vi "Vector Unique Values.vi"(1 "array in":dbl[](array[numeric])) -> (0 "uniques out":dbl[](array[numeric]))   [LabVIEW 2020]
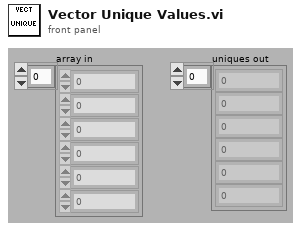
[diagram p1: front panel]
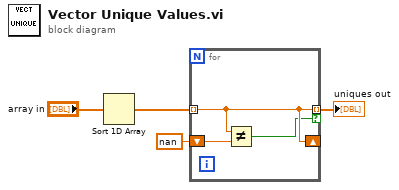
[diagram p0: block diagram]
diagram:
  n1 = Sort 1D Array(array="array in") -> (sorted array=w3:dbl[])
  n2 = for {
    tunnel: w3 -> [w6] mode=indexing
    shift-right: [w6] -> _
    shift-left: nan -> [w7]
    tunnel: [w6] -> w1 mode=indexing if=w5
    n3 = Not Equal?(x=w6, y=w7) -> (x != y?=w5:bool)
  }
  "uniques out" <- w1
